vi "Print.vi"(8 "Error In":errorcluster, 11 "reference in":refnum<class "Menu.lvclass">) -> (0 "Error Out":errorcluster, 3 "reference in":refnum<class "Menu.lvclass">)   [LabVIEW 2020, in "Menu.lvclass"]
uses:
  Menu.lvclass
  MenuComponent_class/MenuComponent.lvclass
  Console_class/Console.lvclass
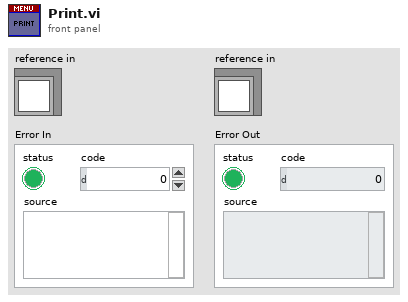
[diagram p1: front panel]
types:
  T1 = typedef "Menu.lvclass/ObjectAttributes.ctl" = cluster{"Items":refnum<class "MenuComponent.lvclass">[], "Name":string, "Description":string}
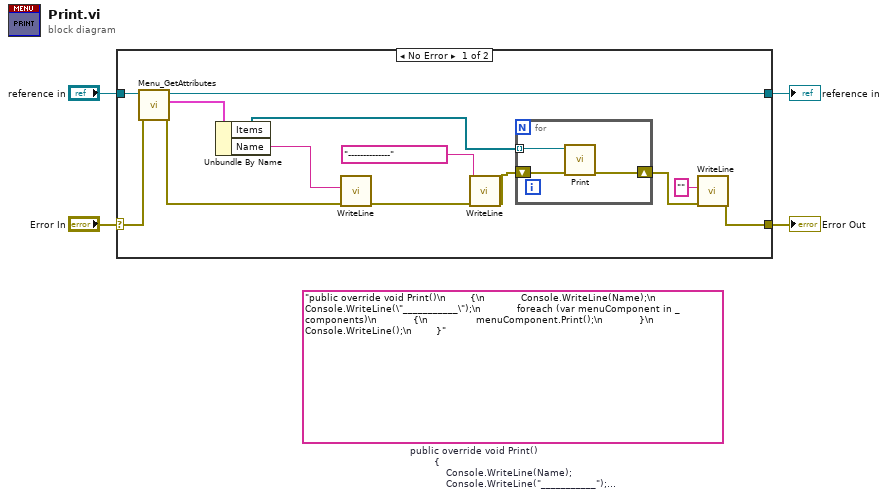
[diagram p0: block diagram]
diagram:
  (unwired) "public override void Print()\n        {\n            Console.WriteLine(Name);\n            Console.WriteLine(\"___________\");\n            foreach (var menuComponent in _components)\n            {\n                menuComponent.Print();\n            }\n            Console.WriteLine();\n        }"  # public override void Print()         {             Console.WriteLine(Name);             Console.WriteLine("___________");             foreach (var menuComponent in _components)             {                 menuComponent.Print();             }             Console.WriteLine();         }
  n1 = case shown="No Error" "Error In" {
    selector: "Error In" -> [w16 w22]
    tunnel: [w6 w22] -> w3
    tunnel: [w15 w21] -> w1
    tunnel: "reference in" -> [w17 w21]
    frame No Error {
      n2 = call "Menu_GetAttributes.vi"("error in (no error)"=w16, "reference in"=w17) -> ("error out"=w11:errorcluster, "Data"=w14:T1, "reference out"=w15:refnum<class "Menu.lvclass">)  [unwired: 6 in, 1 out]
      n3 = Unbundle By Name(w14) -> ("Items"=w13:refnum<class "MenuComponent.lvclass">[], "Name"=w12:string)
      n4 = call "WriteLine.vi"("Error In"=w11, "ConsoleText"=w12) -> ("Error Out"=w10:errorcluster)  [unwired: 9 in]
      n5 = call "WriteLine.vi"("Error In"=w10, "ConsoleText"="--------------") -> ("Error Out"=w8:errorcluster)  [unwired: 9 in]
      n6 = for {
        tunnel: w13 -> [w20] mode=indexing
        shift-right: [w18] -> w7
        shift-left: w8 -> [w19]
        n7 = call-dynamic "Print.vi"("Error In"=w19, "reference in"=w20) -> ("Error Out"=w18:errorcluster)  [unwired: 8 in, 1 out]
      }
      n8 = call "WriteLine.vi"("Error In"=w7, "ConsoleText"="") -> ("Error Out"=w6:errorcluster)  [unwired: 9 in]
    }
    frame Error {
    }
  }
  "Error Out" <- w3
  "reference in" <- w1
